vi "Barrier Attr Get Process.vi"(8 "error in (no error)":errorcluster, 11 "Barrier Attr in":T2) -> (0 "error out":errorcluster, 2 "process":T1, 3 "Barrier Attr out":T2)   [LabVIEW 2016, in "Linux RT IPC.POSIX Threads.lvlib" / "Barrier Attr.lvclass"]
doc: "Calls pthread_barrierattr_getpshared() on the pthread barrier attribute object encapsulated by Barrier Attr.\n\nRefer to online POSIX documentation for more information."
uses:
  Barrier Attr.lvclass
  Controls/reference.ctl
  C:/Git/SourceTree/LinuxRT-IPC/Source/POSIX Threads/Classes/POSIX Thread Object/POSIX Thread Object.lvclass
  Controls/Public/C Enums/pthread_process_shared.ctl
  POSIX Thread Object/POSIX Thread Object.lvclass/POSIX Thread Object.ctl
  POSIX Thread Object/Private VIs/libpthread path.vi
  POSIX Thread Object/Private VIs/get pthread error.vi
  POSIX Thread Object/POSIX Thread Object.lvclass
  Linux RT IPC.POSIX Threads.lvlib
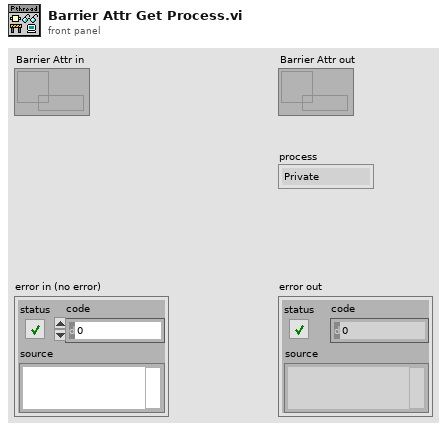
[diagram p1: front panel]
types:
  T1 = typedef "Linux RT IPC.POSIX Threads.lvlib/pthread_process_shared.ctl" = enum16{"Private", "Shared"}
  T2 = typedef "Linux RT IPC.POSIX Threads.lvlib/Barrier Attr.lvclass/reference.ctl" = refnum<data-value>
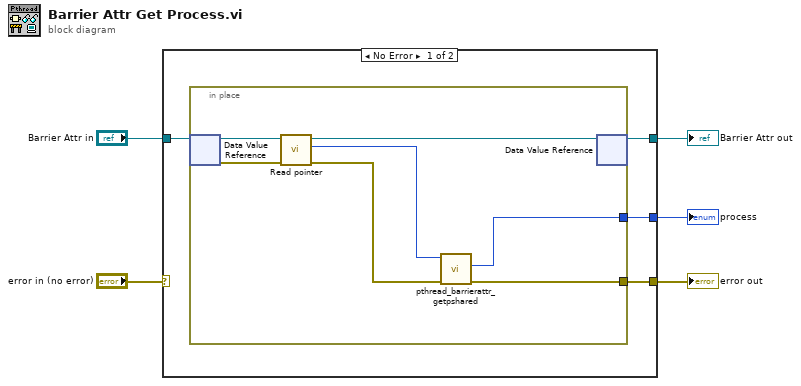
[diagram p0: block diagram]
diagram:
  n1 = case shown="No Error" "error in (no error)" {
    selector: "error in (no error)" -> [_ w18]
    tunnel: [w8 w18] -> w5
    tunnel: [w9 w17] -> w4
    tunnel: "Barrier Attr in" -> [w7 w17]
    tunnel: [w6 _] -> w1
    frame No Error {
      n2 = in-place {
        in-place-border: [w14] -> w8
        in-place-border: [w10] -> w6
        n3 = in-place-dvr #1(w7) -> (w16:refnum<class "Barrier Attr.lvclass">, w12:errorcluster)
        n4 = call "Read pointer.vi"("error in (no error)"=w12, "POSIX Thread Object in"=w16) -> ("error out"=w11:errorcluster, "pointer"=w13:u64, "POSIX Thread Object out"=w15:refnum<class "Barrier Attr.lvclass">)  [unwired: 7 in]
        n5 = call "pthread_barrierattr_getpshared.vi"("error in (no error)"=w11, "barrier attr ptr in"=w13) -> ("error out"=w14:errorcluster, "process shared"=w10:T1)  [unwired: 7 in, 1 out]
        n6 = in-place-dvr #1(w15) -> (w9:T2)  [unwired: 1 out]
      }
    }
    frame Error {
    }
  }
  "Barrier Attr out" <- w4
  "error out" <- w5
  "process" <- w1
